vi "main.vi"() -> ()   [LabVIEW 2014]
uses:
  UI-DisplayTable/UI-DisplayTable(dev).xctl
  UI-DisplayTable/Support/DEF-Filter.ctl
panel:
  out "data":string[](array[string])
  in  "column Value":bool
  in  "Color Box":u32(colorbox)
  in  "reset hightlight":bool
  in  "hightlight":bool
  in  "update lines":bool
  in  "update line":bool
  in  "update":bool
  in  "reset":bool
  in  "delete":bool
  in  "add":bool
  in  "filter":T1
  out "Filter":T1[](array[typedef])
  in  "Column Headers":string[](array[string])=["测试", "һ", "二", "三", "四", "五", "六"]
  in  "Autosize":bool
  in  "Column Widths":i32[](array[numeric])=[64, 64, 64, 64, 64, 64, 64]
  in  "stop":bool
  in  "Max Number":i32=10
  in  "AutoScroll":bool=TRUE
  in  "Add to Top":bool=TRUE
  in  "lines":bool
  in  "line":bool
  in  "AS":i32(xcontrol)
  out "as1":i32=10
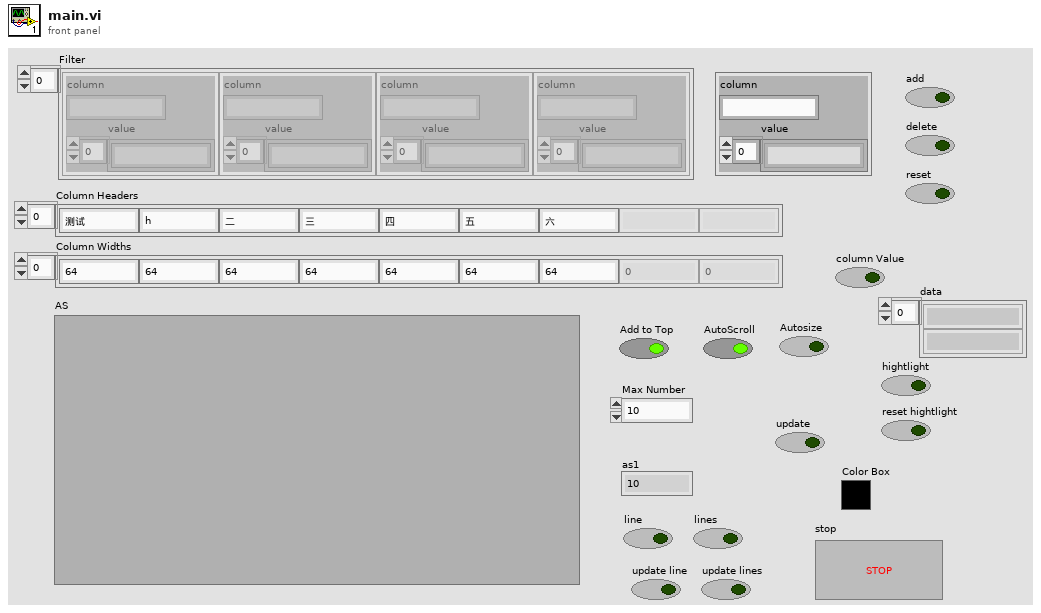
[diagram p1: front panel]
types:
  T1 = typedef "UI-DisplayTable(dev).xctl/DEF-Filter.ctl" = cluster{"column":string, "value":string[]}
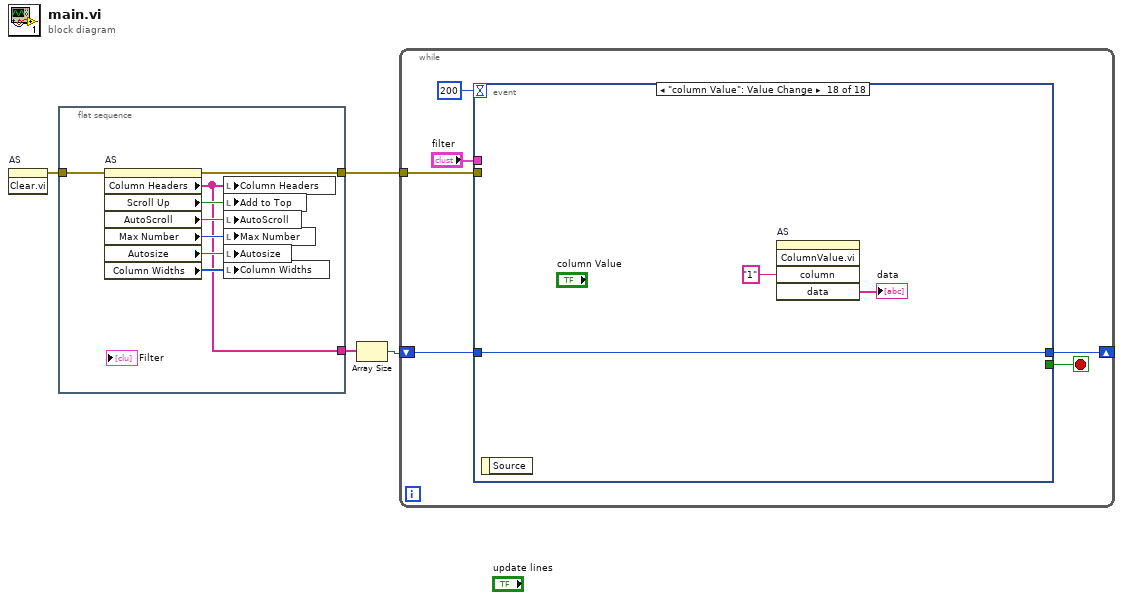
[diagram p0: block diagram]
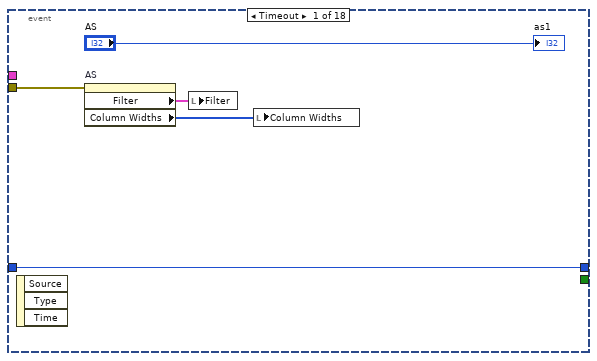
[diagram p2: hidden frame]
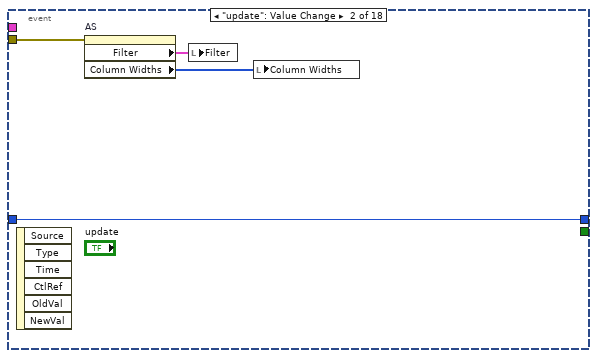
[diagram p3: hidden frame]
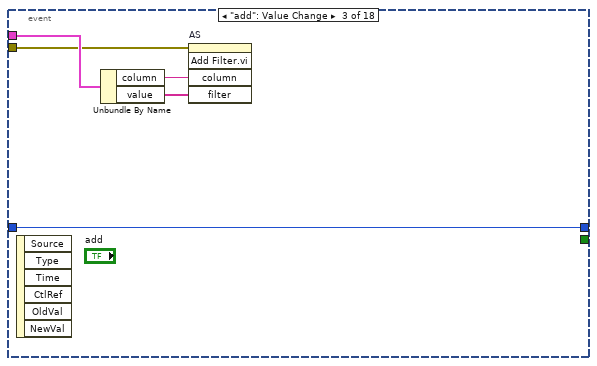
[diagram p4: hidden frame]
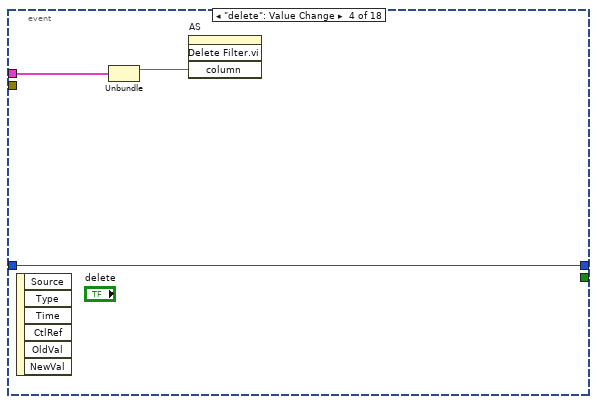
[diagram p5: hidden frame]
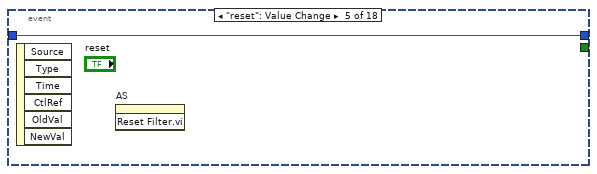
[diagram p6: hidden frame]
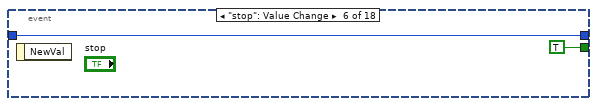
[diagram p7: hidden frame]
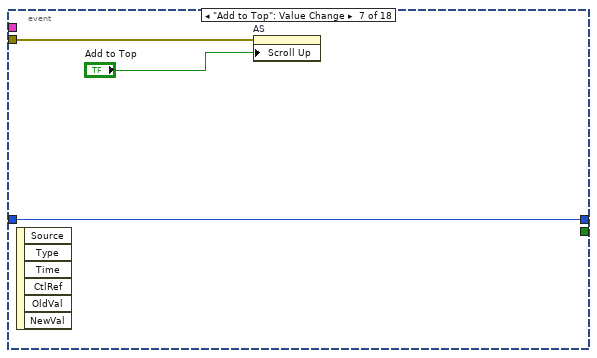
[diagram p8: hidden frame]
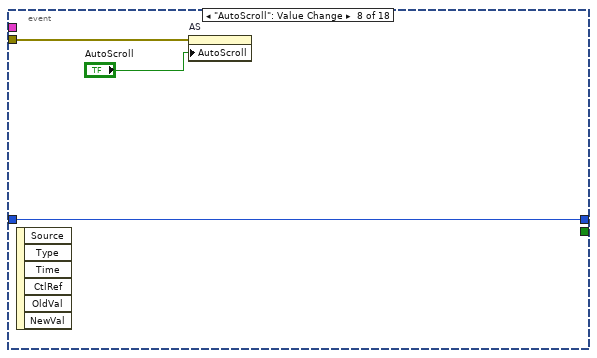
[diagram p9: hidden frame]
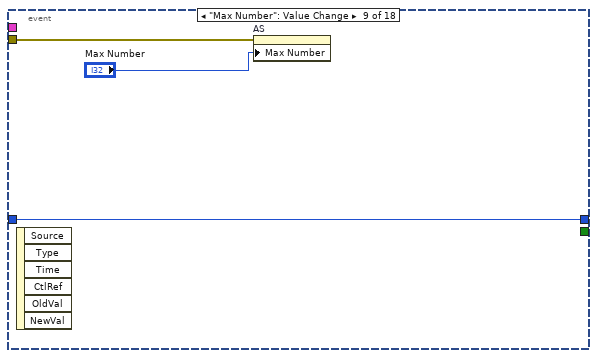
[diagram p10: hidden frame]
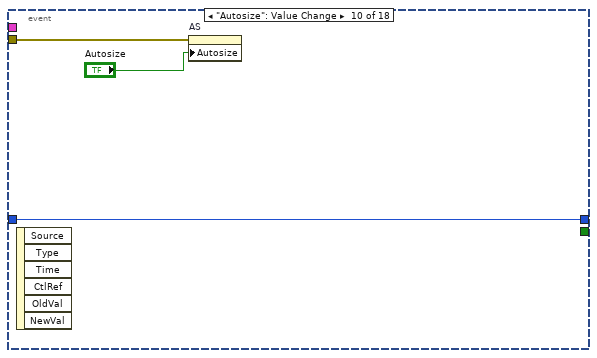
[diagram p11: hidden frame]
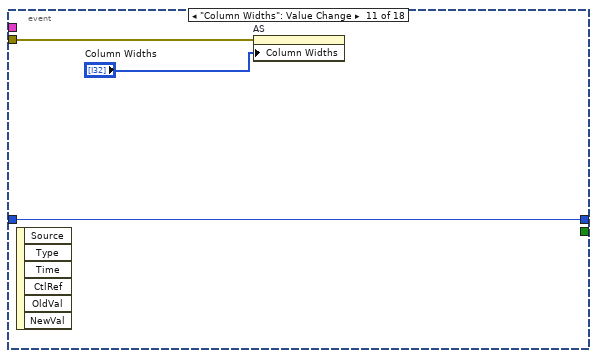
[diagram p12: hidden frame]
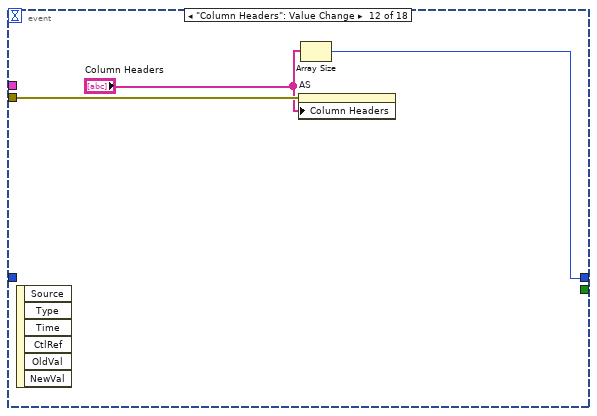
[diagram p13: hidden frame]
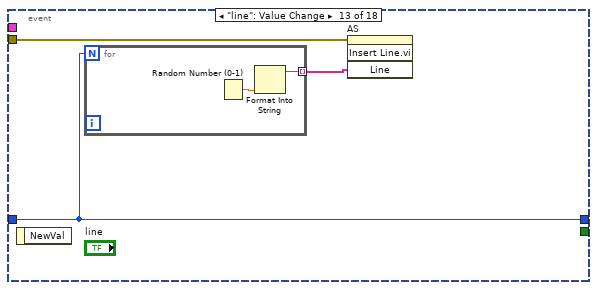
[diagram p14: hidden frame]
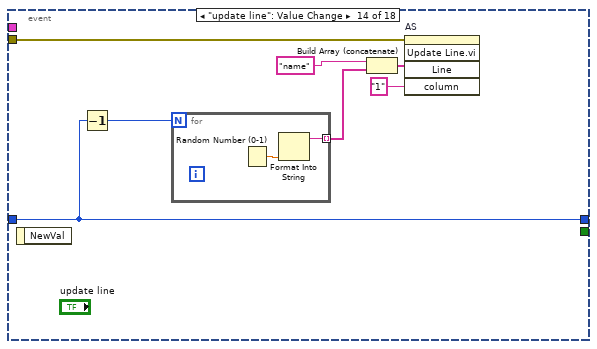
[diagram p15: hidden frame]
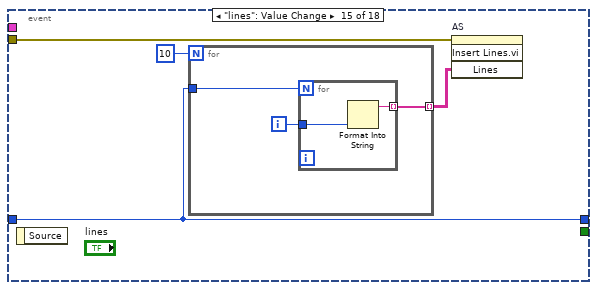
[diagram p16: hidden frame]
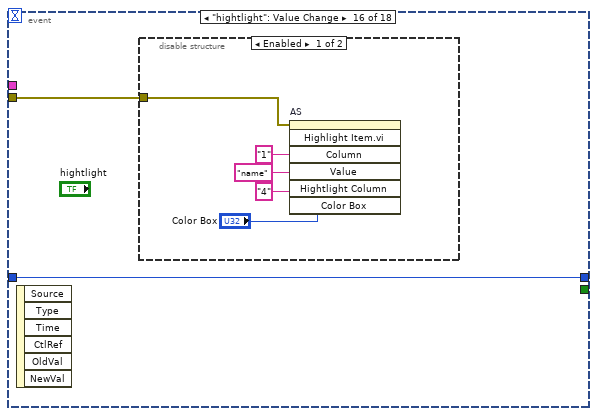
[diagram p17: hidden frame]
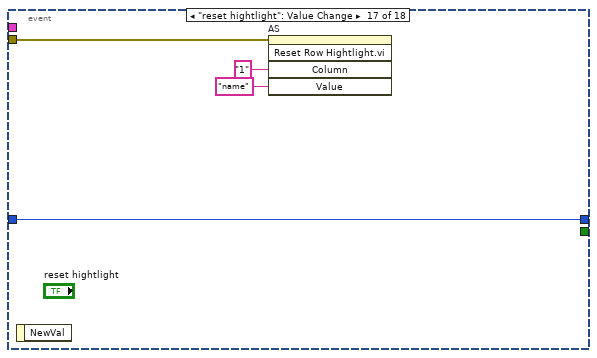
[diagram p19: hidden frame]
diagram:
  n1 = invoke on="AS" class="UI-DisplayTable (strict)" method="Clear.vi"() -> (error out=w3:errorcluster)  [unwired: 3 in, 2 out]
  n2 = flat-sequence {
    tunnel: w3 -> [w12]
    tunnel: [w11] -> w2
    tunnel: [w5] -> w1
    frame #0 {
      n3 = property on="AS" class="UI-DisplayTable(dev) (strict)"(error in=w12) -> (error out=w11:errorcluster, "Column Headers"=w5:string[], "Scroll Up"=w6:bool, "AutoScroll"=w7:bool, "Max Number"=w8:i32, "Autosize"=w9:bool, "Column Widths"=w10:i32[])  [unwired: 1 in, 1 out]
      n4 = local write "Column Headers"(w5) -> ()
      n5 = local write "Add to Top"(w6) -> ()
      n6 = local write "AutoScroll"(w7) -> ()
      n7 = local write "Max Number"(w8) -> ()
      n8 = local write "Autosize"(w9) -> ()
      n9 = local write "Column Widths"(w10) -> ()
    }
  }
  n10 = Array Size(array=w1) -> (size(s)=w4:i32)
  n11 = while {
    tunnel: w2 -> [w16]
    shift-right: [w15] -> _
    shift-left: w4 -> [w17]
    stop <- w18 stop-if-true
    n12 = event shown="[17] \"column Value\": Value Change" {
      selector: _ -> [_ _ _ _ _ _ _ _ _ _ _ _ _ _ _ _ _ _]
      dyn-events: _ -> [_ _ _ _ _ _ _ _ _ _ _ _ _ _ _ _ _ _]
      timeout: 200 -> [_ _ _ _ _ _ _ _ _ _ _ _ _ _ _ _ _ _]
      tunnel: [_ _ _ _ _ TRUE _ _ _ _ _ _ _ _ _ _ _ _] -> w18
      tunnel: w17 -> [w23 w27 w32 w35 w36 w37 w40 w43 w46 w49 w53 _ w58 w67 w74 w81 w90 w93]
      tunnel: w16 -> [w19 w24 w28 _ _ _ w39 w42 w45 w48 w52 w56 w59 w68 w73 w80 w89 _]
      tunnel: [w23 w27 w32 w35 w36 w37 w40 w43 w46 w49 w53 w54 w58 w67 w74 w81 w90 w93] -> w15
      tunnel: "filter" -> [_ _ w29 w34 _ _ _ _ _ _ _ _ _ _ _ _ _ _]
      event Timeout {
        n13 = event-data() -> ()  [unwired: 1 in, 3 out]
        n14 = property on="AS" class="UI-DisplayTable(dev) (strict)"(error in=w19) -> ("Filter"=w21:T1[], "Column Widths"=w22:i32[])  [unwired: 1 in, 2 out]
        n15 = local write "Filter"(w21) -> ()
        n16 = local write "Column Widths"(w22) -> ()
        "as1" <- "AS"
      }
      event "update": Value Change {
        n17 = event-data() -> ()  [unwired: 1 in, 6 out]
        n18 = property on="AS" class="UI-DisplayTable(dev) (strict)"(error in=w24) -> ("Filter"=w25:T1[], "Column Widths"=w26:i32[])  [unwired: 1 in, 2 out]
        n19 = local write "Filter"(w25) -> ()
        n20 = local write "Column Widths"(w26) -> ()
      }
      event "add": Value Change {
        n21 = event-data() -> ()  [unwired: 1 in, 6 out]
        n22 = Unbundle By Name(w29) -> ("column"=w31:string, "value"=w30:string[])
        n23 = invoke on="AS" class="UI-DisplayTable (strict)" method="Add Filter.vi"(error in=w28, "column"=w31, "filter"=w30) -> ()  [unwired: 2 in, 5 out]
      }
      event "delete": Value Change {
        n24 = event-data() -> ()  [unwired: 1 in, 6 out]
        n25 = Unbundle(w34) -> ("column"=w33:string)  [unwired: 1 out]
        n26 = invoke on="AS" class="UI-DisplayTable (strict)" method="Delete Filter.vi"("column"=w33) -> ()  [unwired: 3 in, 4 out]
      }
      event "reset": Value Change {
        n27 = event-data() -> ()  [unwired: 1 in, 6 out]
        n28 = invoke on="AS" class="UI-DisplayTable (strict)" method="Reset Filter.vi"() -> ()  [unwired: 3 in, 3 out]
      }
      event "stop": Value Change {
        n29 = event-data() -> ()  [unwired: 1 in, 1 out]
      }
      event "Add to Top": Value Change {
        n30 = event-data() -> ()  [unwired: 1 in, 6 out]
        n31 = property on="AS" class="UI-DisplayTable(dev) (strict)"(error in=w39, "Scroll Up"="Add to Top") -> ()  [unwired: 1 in, 2 out]
      }
      event "AutoScroll": Value Change {
        n32 = event-data() -> ()  [unwired: 1 in, 6 out]
        n33 = property on="AS" class="UI-DisplayTable(dev) (strict)"(error in=w42, "AutoScroll"="AutoScroll") -> ()  [unwired: 1 in, 2 out]
      }
      event "Max Number": Value Change {
        n34 = event-data() -> ()  [unwired: 1 in, 6 out]
        n35 = property on="AS" class="UI-DisplayTable(dev) (strict)"(error in=w45, "Max Number"="Max Number") -> ()  [unwired: 1 in, 2 out]
      }
      event "Autosize": Value Change {
        n36 = event-data() -> ()  [unwired: 1 in, 6 out]
        n37 = property on="AS" class="UI-DisplayTable(dev) (strict)"(error in=w48, "Autosize"="Autosize") -> ()  [unwired: 1 in, 2 out]
      }
      event "Column Widths": Value Change {
        n38 = event-data() -> ()  [unwired: 1 in, 6 out]
        n39 = property on="AS" class="UI-DisplayTable(dev) (strict)"(error in=w52, "Column Widths"="Column Widths") -> ()  [unwired: 1 in, 2 out]
      }
      event "Column Headers": Value Change {
        n40 = event-data() -> ()  [unwired: 1 in, 6 out]
        n41 = property on="AS" class="UI-DisplayTable(dev) (strict)"(error in=w56, "Column Headers"="Column Headers") -> ()  [unwired: 1 in, 2 out]
        n42 = Array Size(array="Column Headers") -> (size(s)=w54:i32)
      }
      event "line": Value Change {
        n43 = event-data() -> ()  [unwired: 1 in, 1 out]
        n44 = for {
          N: w58 -> [_]
          tunnel: [w60] -> w57 mode=indexing
          n45 = Random Number (0-1)() -> (number: 0 to 1=w61:dbl)
          n46 = Format Into String(w61) -> (resulting string=w60:string)  [unwired: 3 in, 1 out]
        }
        n47 = invoke on="AS" class="UI-DisplayTable (strict)" method="Insert Line.vi"(error in=w59, "Line"=w57) -> ()  [unwired: 2 in, 4 out]
      }
      event "update line": Value Change {
        n48 = event-data() -> ()  [unwired: 1 in, 1 out]
        n49 = Decrement(x=w67) -> (x-1=w65:i32)
        n50 = for {
          N: w65 -> [_]
          tunnel: [w69] -> w66 mode=indexing
          n51 = Random Number (0-1)() -> (number: 0 to 1=w70:dbl)
          n52 = Format Into String(w70) -> (resulting string=w69:string)  [unwired: 3 in, 1 out]
        }
        n53 = Build Array (concatenate)("name" ("column"), w66) -> (w63:string[])
        n54 = invoke on="AS" class="UI-DisplayTable (strict)" method="Update Line.vi"(error in=w68, "Line"=w63, "column"="1") -> ()  [unwired: 2 in, 5 out]
      }
      event "lines": Value Change {
        n55 = event-data() -> ()  [unwired: 1 in, 1 out]
        n56 = for {
          N: 10 -> [_]
          tunnel: [w77] -> w72 mode=indexing
          tunnel: w74 -> [w76]
          i -> [w75]
          n57 = for {
            N: w76 -> [_]
            tunnel: [w79] -> w77 mode=indexing
            tunnel: w75 -> [w78]
            n58 = Format Into String(w78) -> (resulting string=w79:string)  [unwired: 3 in, 1 out]
          }
        }
        n59 = invoke on="AS" class="UI-DisplayTable (strict)" method="Insert Lines.vi"(error in=w73, "Lines"=w72) -> ()  [unwired: 2 in, 4 out]
      }
      event "hightlight": Value Change {
        n60 = event-data() -> ()  [unwired: 1 in, 6 out]
        n61 = disable-structure shown="Enabled" {
          disable-tunnel: w80 -> [w86 _]
          frame Enabled {
            n62 = invoke on="AS" class="UI-DisplayTable (strict)" method="Highlight Item.vi"(error in=w86, "Column"="1", "Value"="name", "Hightlight Column"="4", "Color Box"="Color Box") -> ()  [unwired: 2 in, 7 out]
          }
          frame Disabled {
          }
        }
      }
      event "reset hightlight": Value Change {
        n63 = event-data() -> ()  [unwired: 1 in, 1 out]
        n64 = invoke on="AS" class="UI-DisplayTable (strict)" method="Reset Row Hightlight.vi"(error in=w89, "Column"="1", "Value"="name") -> ()  [unwired: 2 in, 5 out]
      }
      event "column Value": Value Change {
        n65 = event-data() -> ()  [unwired: 1 in, 1 out]
        n66 = invoke on="AS" class="UI-DisplayTable (strict)" method="ColumnValue.vi"("column"="1") -> ("data"=→"data":string[])  [unwired: 4 in, 4 out]
      }
    }
  }
